vi "converte_signal_to_phy_value.vi"(10 "data in":dbl[](array[numeric])) -> (2 "data out":dbl[](array[numeric]))   [LabVIEW 2020]
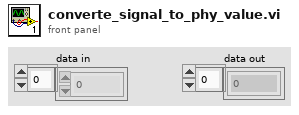
[diagram p1: front panel]
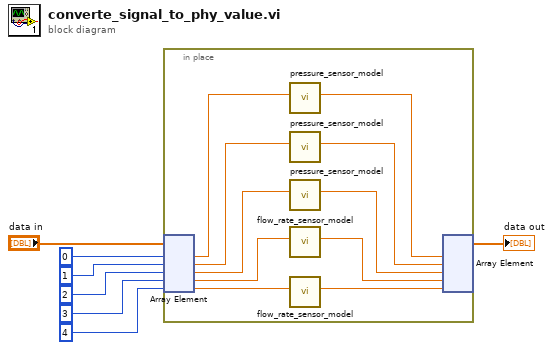
[diagram p0: block diagram]
diagram:
  n1 = in-place {
    n2 = in-place-array #1("data in", 0, 1, 2, 3, 4) -> (w17:dbl, w16:dbl, w15:dbl, w14:dbl, w13:dbl)
    n3 = call "pressure_sensor_model.vi"("input(A)"=w17) -> ("output(bar)"=w12:dbl)  [unwired: 10 in]
    n4 = call "pressure_sensor_model.vi"("input(A)"=w16) -> ("output(bar)"=w11:dbl)  [unwired: 10 in]
    n5 = call "pressure_sensor_model.vi"("input(A)"=w15) -> ("output(bar)"=w10:dbl)  [unwired: 10 in]
    n6 = call "flow_rate_sensor_model.vi"("input(A)"=w14) -> ("output(LPM)"=w9:dbl)  [unwired: 10 in]
    n7 = call "flow_rate_sensor_model.vi"("input(A)"=w13) -> ("output(LPM)"=w8:dbl)  [unwired: 10 in]
    n8 = in-place-array #1(w12, w11, w10, w9, w8) -> (→"data out":dbl[])  [unwired: 5 out]
  }
